vi "Main.vi"(8 "error":errorcluster) -> (0 "Error out":errorcluster)   [LabVIEW 2018, in "GUI3.lvclass"]
uses:
  GUI3.lvclass
  Public Controls/TestInfo.ctl
  S6/S6.lvclass
  S5/S5.lvclass
panel:
  in  "Tab Control":enum32{"TESTS SCREEN"}(tab)
  out "S5 Valves":bool[](array[boolean])
  out "EC_PTEST_DELTA_MAX":dbl format="%.2f psig"
  in  "S5AckAlarm":bool
  out "PRESSURE PT1_S6":dbl(knob) caption="PRESSURE PT1" scale=0.0..400.0
  out "ELAPSED TIME 5":dbl caption="REMAINING STATE TIME" format="%<%H:%M:%S>t"
  out "IsLidLocked_S5":bool caption="IsLidLocked"
  in  "SN_S5":string caption="SN"
  in  "S5Start":bool
  in  "ABORT_S5":bool
  out "TEST STOPPED AT:":string
  out "TEST STARTED AT:":string
  out "PRESSURE PT531":dbl(knob) scale=0.0..400.0
  out "PRESSURE PT521":dbl(knob) scale=0.0..400.0
  out "TEST RESULT_S5":string caption="TEST RESULT"
  out "TEST STATE_S5":string caption="TEST STATE"
  out "Pressure vs Time Plot 3":waveform(dbl)[](graph)
  out "TEST STATUS 5":string caption="TEST STATUS"
  in  "Select Test Type_S5":string(combo) caption="Test Type"
  out "S6 Valves":bool[](array[boolean])
  out "EC_PTEST_DELTA_MAX":dbl format="%.2f psig"
  in  "S6AckAlarm":bool
  out "PRESSURE PT1_S5":dbl(knob) caption="PRESSURE PT1" scale=0.0..400.0
  out "ELAPSED TIME 6":dbl caption="REMAINING STATE TIME" format="%<%H:%M:%S>t"
  out "IsLidLocked_S6":bool caption="IsLidLocked"
  in  "SN_S6":string caption="SN"
  in  "S6Start":bool
  in  "ABORT_S6":bool
  out "TEST STOPPED AT:":string
  out "TEST STARTED AT:":string
  out "PRESSURE PT631":dbl(knob) scale=0.0..400.0
  out "PRESSURE PT621":dbl(knob) scale=0.0..400.0
  out "TEST RESULT_S6":string caption="TEST RESULT"
  out "TEST STATE_S6":string caption="TEST STATE"
  out "Pressure vs Time Plot 4":waveform(dbl)[](graph)
  out "TEST STATUS 6":string caption="TEST STATUS"
  in  "Select Test Type_S6":string(combo) caption="Test Type"
  # "This template is for the Simple State Machine design pattern.\n\nSee the block diagram for more information on how to use this template."
  # "STATION #5"
  # "STATION #6"
  # "LoP"
  # "HiP"
  # "Z3"
  # "Z2"
  # "Lid Ext"
  # "LoP"
  # "HiP"
  # "Z3"
  # "Z2"
  # "Lid Ext"
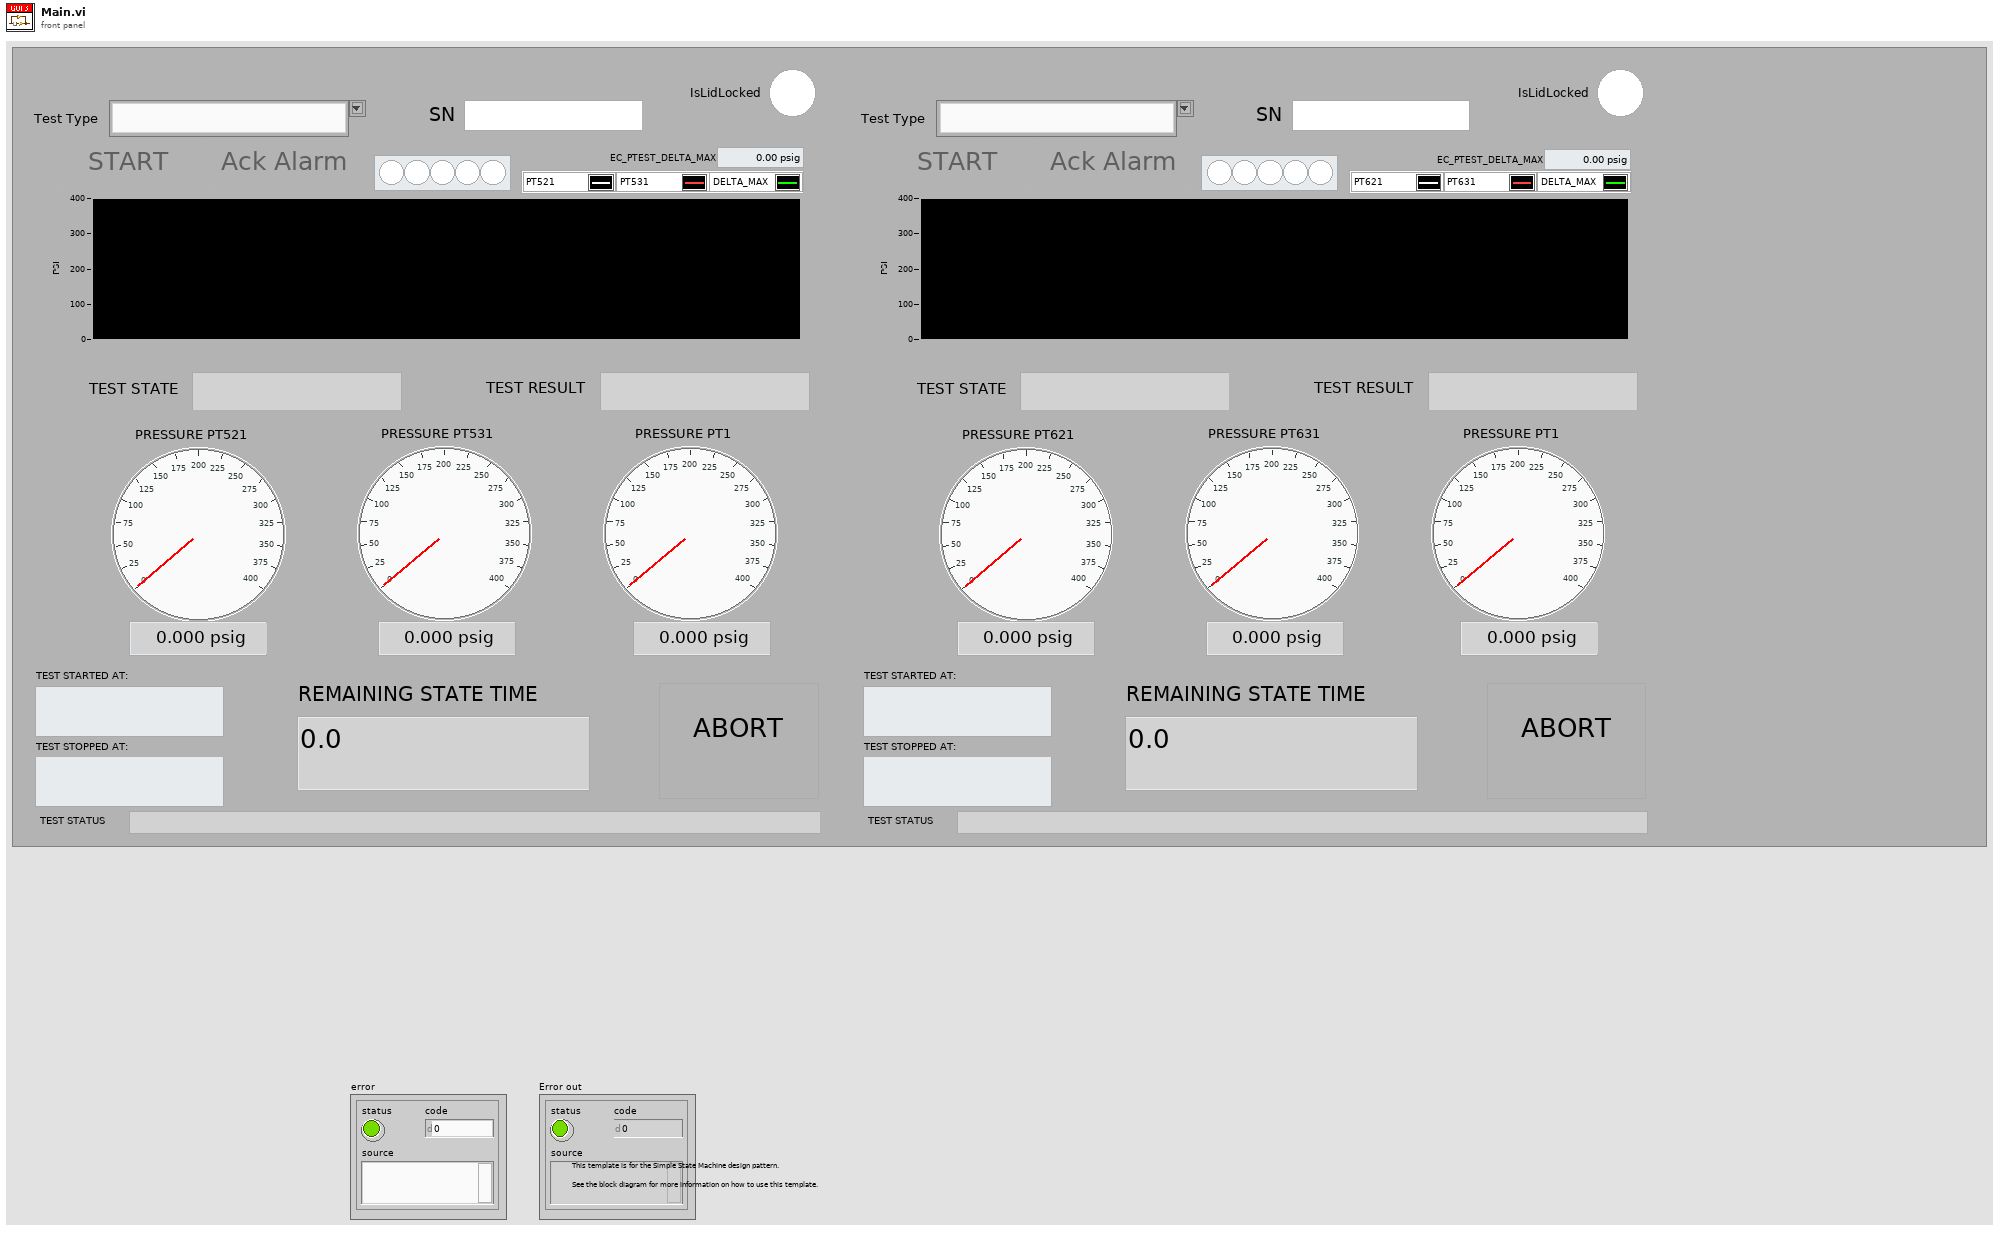
[diagram p1: front panel]
types:
  T1 = enum8{"Enabled", "Disabled", "Disabled and Grayed Out"}
  T2 = typedef "GUI3.lvclass/State.ctl" = enum16{"Initialize", "S5Alarm", "S6Alarm", "S5EndOfTest", "S6EndOfTest", "Monitor", "Error", "Exit"}
  T3 = typedef "GUI3.lvclass/TestInfo.ctl" = cluster{"TestType":string, "SN":string}
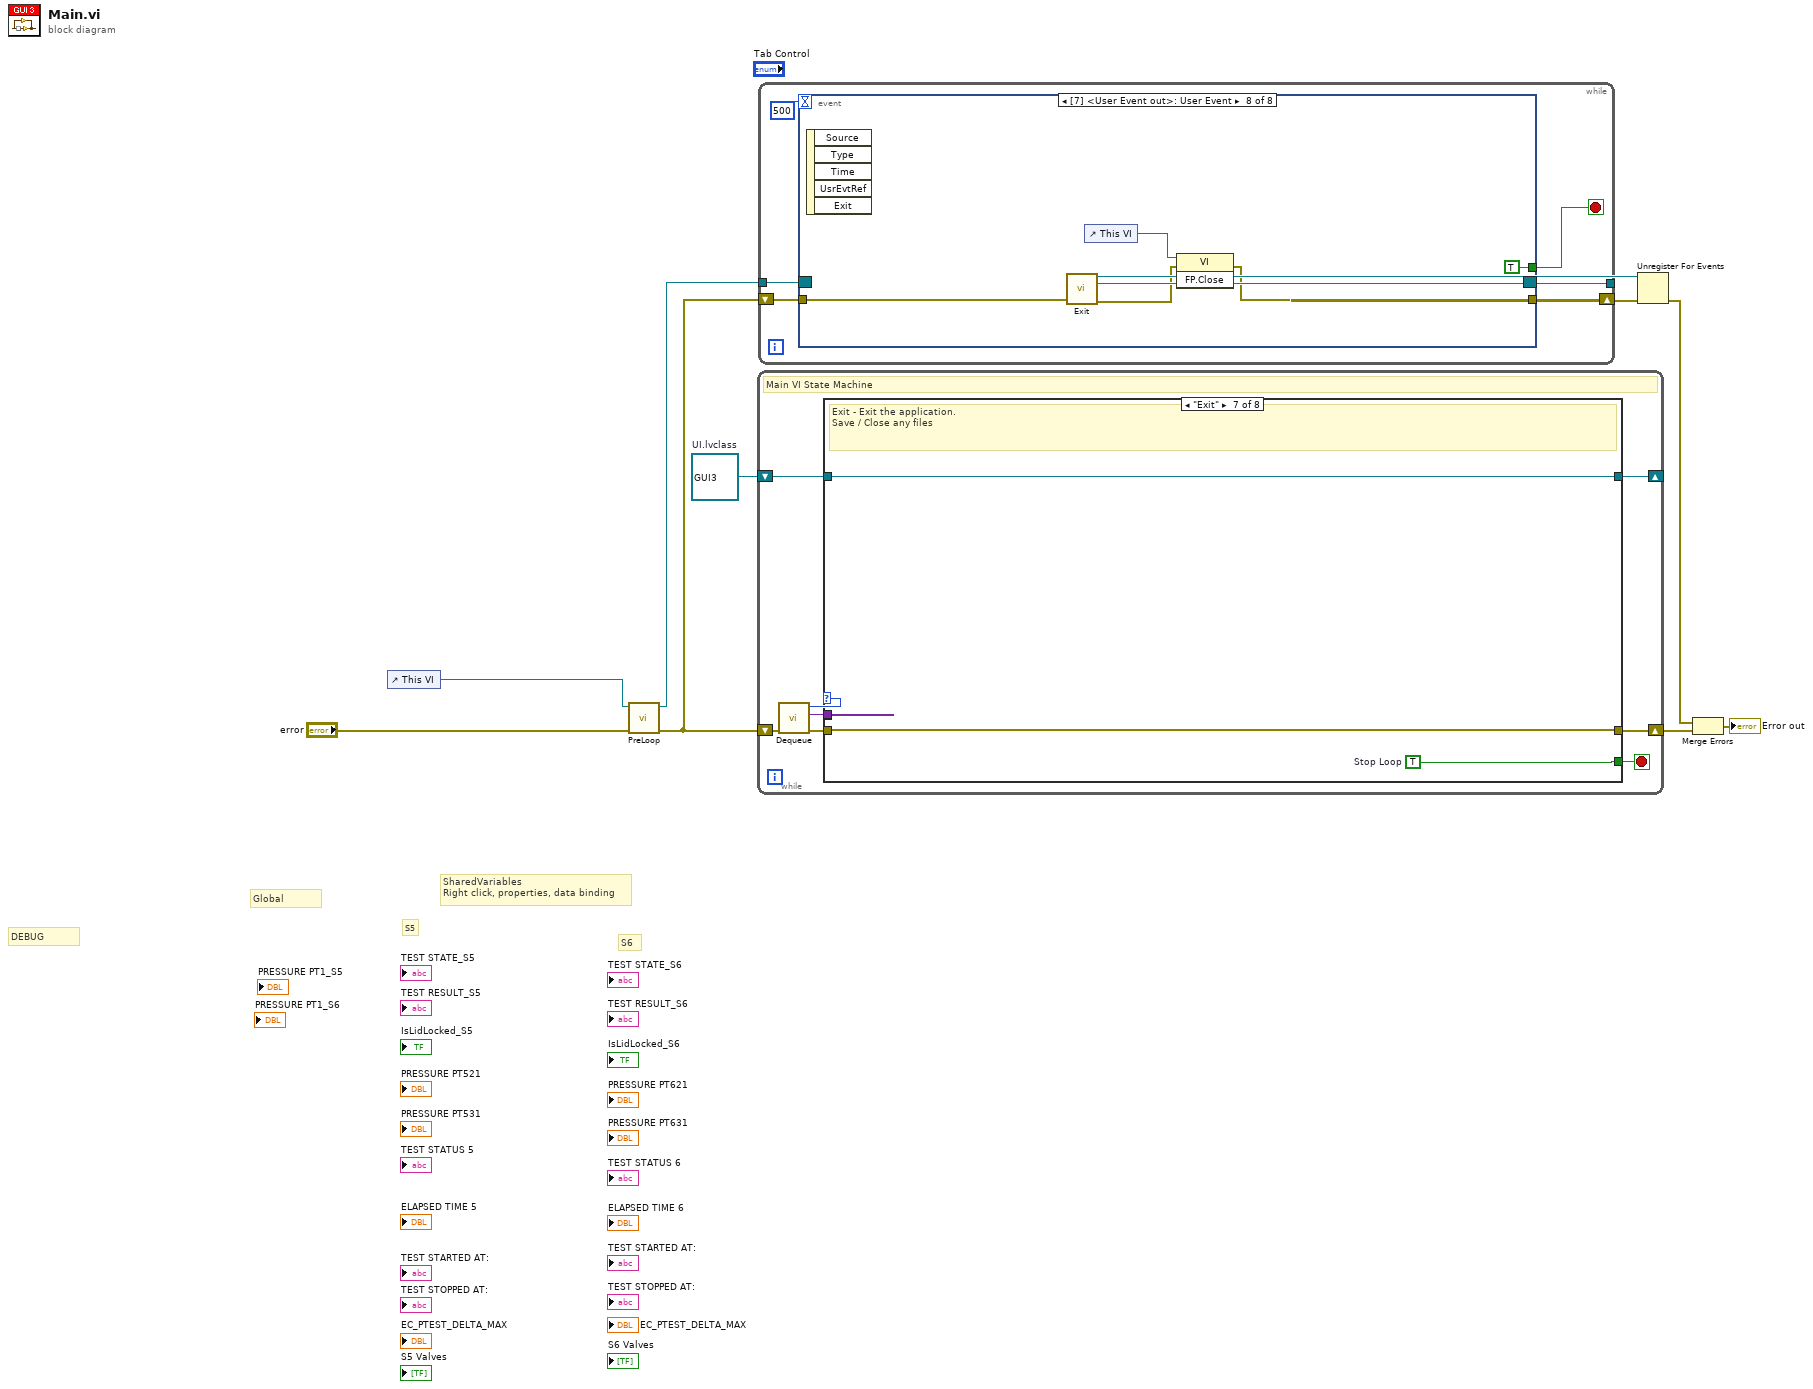
[diagram p0: block diagram]
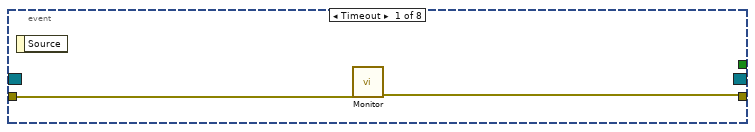
[diagram p2: hidden frame]
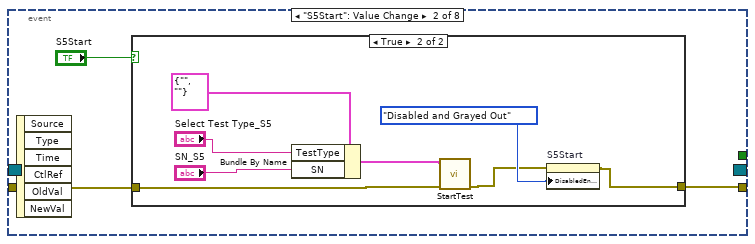
[diagram p3: hidden frame]
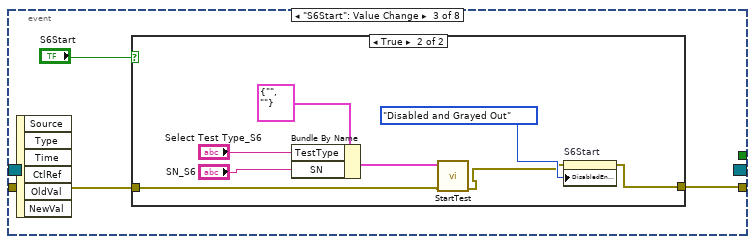
[diagram p5: hidden frame]
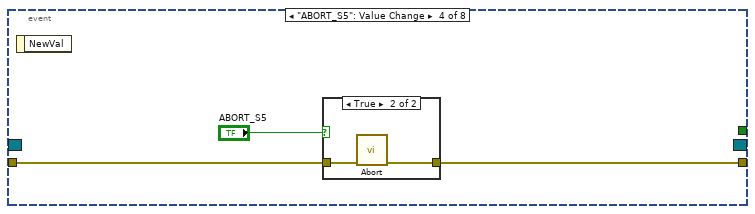
[diagram p7: hidden frame]
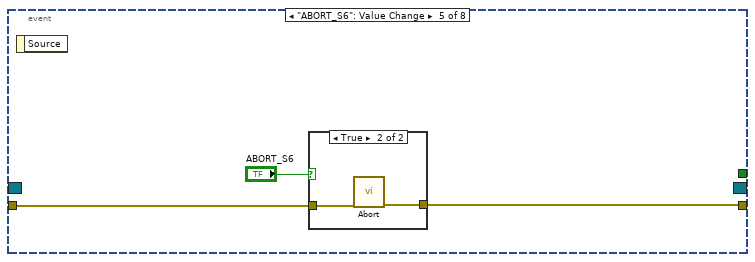
[diagram p9: hidden frame]
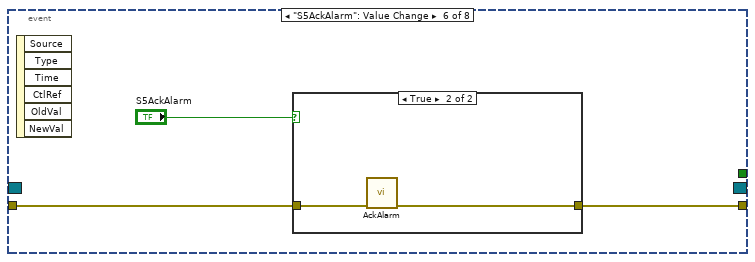
[diagram p11: hidden frame]
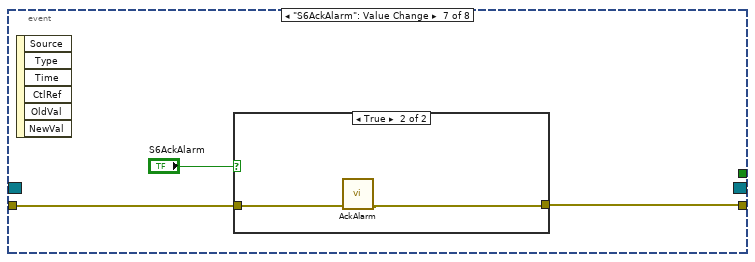
[diagram p13: hidden frame]
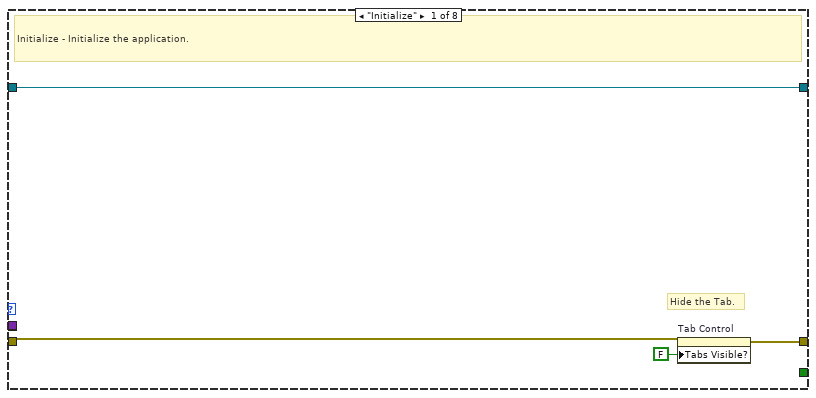
[diagram p15: hidden frame]
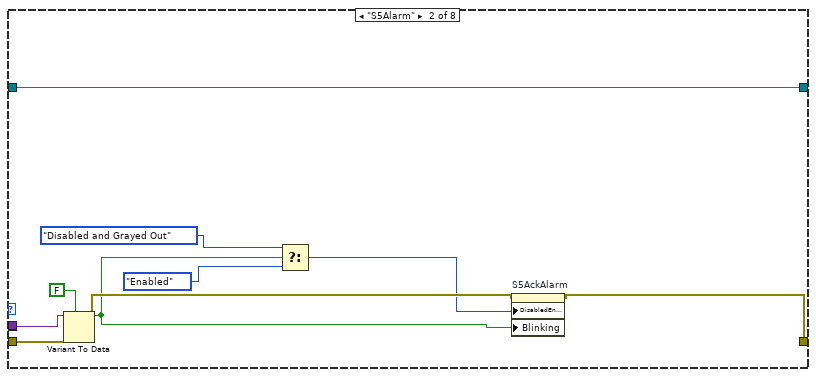
[diagram p16: hidden frame]
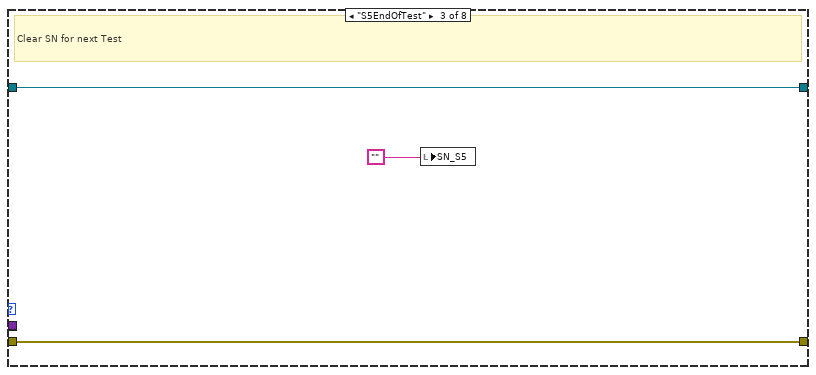
[diagram p17: hidden frame]
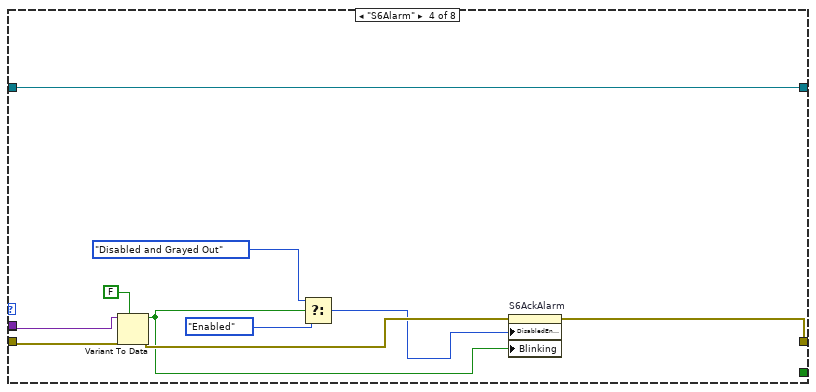
[diagram p18: hidden frame]
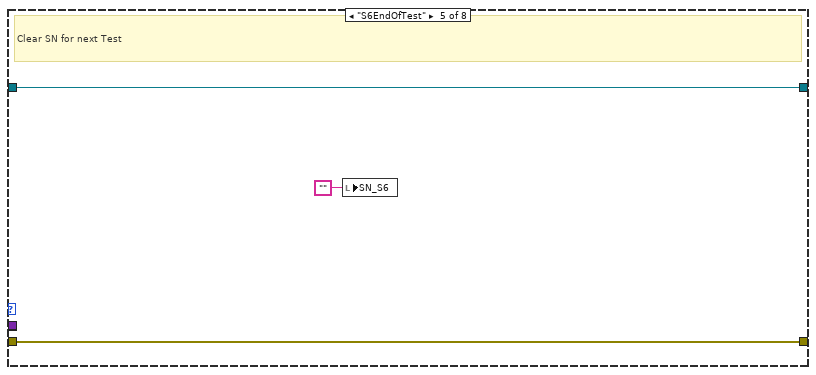
[diagram p19: hidden frame]
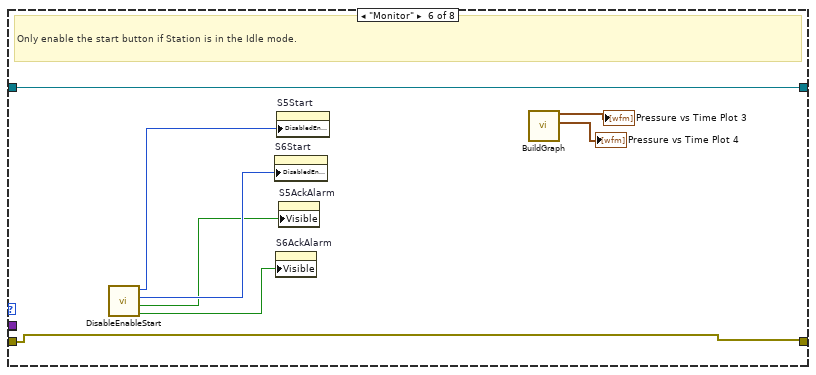
[diagram p20: hidden frame]
diagram:
  w10 = refnum<class "GUI3.lvclass"> refnum  # UI.lvclass
  # "Global"
  # "S6"
  # "DEBUG"
  # "S5"
  # "SharedVariables\nRight click, properties, data binding"
  n1 = control-ref of="This VI"() -> (w1:refnum<vi>)
  n2 = call "PreLoop.vi"("error in"="error", "VI Ref"=w1) -> ("error out"=w9:errorcluster, "Event Out"=w3:refnum<event-registration>)  [unwired: 8 in]
  n3 = while {
    shift-right: [w18] -> w6
    shift-left: w9 -> [w14]
    shift-right: [w15] -> _
    shift-left: w10 -> [w16]
    stop <- w17 stop-if-true
    # "Main VI State Machine"
    n4 = call "Dequeue.vi"("error in"=w14) -> ("error out"=w13:errorcluster, "Data"=w11:variant, "State"=w12:T2)  [unwired: 8 in]
    n5 = case shown="\"Exit\"" w12 {
      tunnel: [_ _ _ _ _ _ w59 _] -> w17
      tunnel: w13 -> [w19 w31 w35 w41 w48 w49 w57 w65]
      tunnel: [w20 w25 w35 w36 w48 w49 w57 w61] -> w18
      tunnel: w16 -> [w22 w32 w34 w45 w47 w56 w58 w68]
      tunnel: [w22 w32 w34 w45 w47 w56 w58 w68] -> w15
      tunnel: w11 -> [_ w30 _ w40 _ _ _ w64]
      tunnel: w11 -> [_ _ _ _ _ _ _ _]
      frame "Initialize" {
        # "Hide the Tab."
        # "Initialize - Initialize the application."
        n6 = property on="Tab Control" class="TabCtl (strict)"(error in=w19, "Tabs Visible?"=FALSE) -> (error out=w20:errorcluster)  [unwired: 1 in, 1 out]
      }
      frame "S5Alarm" {
        n7 = Variant To Data(error in=w31, type=FALSE, Variant=w30) -> (data=w23:bool, error out=w26:errorcluster)
        n8 = Select(t=T1."Disabled and Grayed Out" ("Disabled"), s=w23, f=T1."Enabled" ("Disabled")) -> (s? t:f=w24:T1)
        n9 = property on="S5AckAlarm" class="Bool"(error in=w26, "DisabledEnum"=w24, "Blinking"=w23) -> (error out=w25:errorcluster)  [unwired: 1 in, 1 out]
      }
      frame "S5EndOfTest" {
        # "Clear SN for next Test"
        n10 = local write "SN_S5"("" ("SN")) -> ()
      }
      frame "S6Alarm" {
        n11 = Variant To Data(error in=w41, type=FALSE, Variant=w40) -> (data=w37:bool, error out=w39:errorcluster)
        n12 = Select(t=T1."Disabled and Grayed Out" ("Disabled"), s=w37, f=T1."Enabled" ("Disabled")) -> (s? t:f=w38:T1)
        n13 = property on="S6AckAlarm" class="Bool"(error in=w39, "DisabledEnum"=w38, "Blinking"=w37) -> (error out=w36:errorcluster)  [unwired: 1 in, 1 out]
      }
      frame "S6EndOfTest" {
        # "Clear SN for next Test"
        n14 = local write "SN_S6"("") -> ()
      }
      frame "Monitor" {
        # "Only enable the start button if Station is in the Idle mode."
        n15 = call "DisableEnableStart.vi"() -> ("S6AckVisable"=w50:bool, "S5AckVisable"=w52:bool, "Station6"=w55:T1, "Station5"=w51:T1)  [unwired: 8 in]
        n16 = property on="S6Start" class="Bool"("DisabledEnum"=w55) -> ()  [unwired: 2 in, 2 out]
        n17 = property on="S6AckAlarm" class="Bool"("Visible"=w50) -> ()  [unwired: 2 in, 2 out]
        n18 = property on="S5Start" class="Bool"("DisabledEnum"=w51) -> ()  [unwired: 2 in, 2 out]
        n19 = property on="S5AckAlarm" class="Bool"("Visible"=w52) -> ()  [unwired: 2 in, 2 out]
        n20 = call "BuildGraph.vi"() -> ("S6"=→"Pressure vs Time Plot 4":waveform(dbl)[], "S5"=→"Pressure vs Time Plot 3":waveform(dbl)[])  [unwired: 10 in]
      }
      frame "Exit" {
        w59 = TRUE  # Stop Loop
        # "Exit - Exit the application.\nSave / Close any files"
      }
      frame "Error" {
        n21 = Variant To Data(error in=w65, type=errorcluster {"status"=FALSE, "code"=0, "source"=""} ("error out"), Variant=w64) -> (data=w66:errorcluster, error out=w62:errorcluster)
        n22 = Unbundle By Name(w66) -> ("code"=w60:i32, "source"=w63:string)
        n23 = case shown="Default" w60 {
          tunnel: w63 -> [_ w71]
          tunnel: w62 -> [w69 w73]
          tunnel: [w69 w73] -> w61
          frame 1 {
            # "Error talking to other modules. \n\nIgnore. If testing by itself."
          }
          frame Default {
            n24 = Concatenate Strings("Error on GUI" ("message"), w71) -> (w70:string)
            n25 = One Button Dialog(message=w70) -> ()  [unwired: 1 in, 1 out]
          }
        }
      }
    }
  }
  n26 = while {
    shift-right: [w77] -> w8
    shift-left: w9 -> [w79]
    tunnel: [w76] -> w7
    tunnel: w3 -> [w74]
    stop <- w78 stop-if-true
    n27 = event shown="[7] <User Event out>: User Event" {
      selector: w74 -> [_ _ _ _ _ _ _ _]
      dyn-events: [_ _ _ _ _ _ _ _] -> w76
      timeout: 500 -> [_ _ _ _ _ _ _ _]
      tunnel: w79 -> [w81 w84 w96 w108 w114 w120 w125 w134]
      tunnel: [w80 w83 w95 w107 w112 w119 w124 w130] -> w77
      tunnel: [_ _ _ _ _ _ _ TRUE] -> w78
      event Timeout {
        n28 = event-data() -> ()  [unwired: 1 in, 1 out]
        n29 = call "Monitor.vi"("error in"=w81) -> ("error out"=w80:errorcluster)  [unwired: 10 in]
      }
      event "S5Start": Value Change {
        n30 = event-data() -> ()  [unwired: 1 in, 6 out]
        n31 = case shown="True" "S5Start" {
          tunnel: w84 -> [w85 w87]
          tunnel: [w85 w89] -> w83
          frame False {
          }
          frame True {
            n32 = Bundle By Name(cluster=T3 {"TestType"="", "SN"=""}, "TestType"="Select Test Type_S5", "SN"="SN_S5") -> (w88:T3)
            n33 = call "StartTest.vi"("error in"=w87, "TestInfo"=w88) -> ("error out"=w86:errorcluster)  [unwired: 9 in]
            n34 = property on="S5Start" class="Bool"(error in=w86, "DisabledEnum"=T1."Disabled and Grayed Out" ("Disabled")) -> (error out=w89:errorcluster)  [unwired: 1 in, 1 out]
          }
        }
      }
      event "S6Start": Value Change {
        n35 = event-data() -> ()  [unwired: 1 in, 6 out]
        n36 = case shown="True" "S6Start" {
          tunnel: w96 -> [w97 w99]
          tunnel: [w97 w102] -> w95
          frame False {
          }
          frame True {
            n37 = Bundle By Name(cluster=T3 {"TestType"="", "SN"=""}, "TestType"="Select Test Type_S6", "SN"="SN_S6") -> (w100:T3)
            n38 = call "StartTest.vi"("error in"=w99, "TestInfo"=w100) -> ("error out"=w98:errorcluster)  [unwired: 9 in]
            n39 = property on="S6Start" class="Bool"(error in=w98, "DisabledEnum"=T1."Disabled and Grayed Out" ("Disabled")) -> (error out=w102:errorcluster)  [unwired: 1 in, 1 out]
          }
        }
      }
      event "ABORT_S5": Value Change {
        n40 = event-data() -> ()  [unwired: 1 in, 1 out]
        n41 = case shown="True" "ABORT_S5" {
          tunnel: w108 -> [w109 w111]
          tunnel: [w109 w110] -> w107
          frame False {
          }
          frame True {
            n42 = call "Abort.vi"("error in"=w111) -> ("error out"=w110:errorcluster)  [unwired: 10 in]
          }
        }
      }
      event "ABORT_S6": Value Change {
        n43 = event-data() -> ()  [unwired: 1 in, 1 out]
        n44 = case shown="True" "ABORT_S6" {
          tunnel: w114 -> [w115 w117]
          tunnel: [w115 w116] -> w112
          frame False {
          }
          frame True {
            n45 = call "Abort.vi"("error in"=w117) -> ("error out"=w116:errorcluster)  [unwired: 10 in]
          }
        }
      }
      event "S5AckAlarm": Value Change {
        n46 = event-data() -> ()  [unwired: 1 in, 6 out]
        n47 = case shown="True" "S5AckAlarm" {
          tunnel: w120 -> [w121 w123]
          tunnel: [w121 w122] -> w119
          frame False {
          }
          frame True {
            n48 = call "AckAlarm.vi"("error in"=w123) -> ("error out"=w122:errorcluster)  [unwired: 10 in]
          }
        }
      }
      event "S6AckAlarm": Value Change {
        n49 = event-data() -> ()  [unwired: 1 in, 6 out]
        n50 = case shown="True" "S6AckAlarm" {
          tunnel: w125 -> [w127 w129]
          tunnel: [w127 w128] -> w124
          frame False {
          }
          frame True {
            n51 = call "AckAlarm.vi"("error in"=w129) -> ("error out"=w128:errorcluster)  [unwired: 10 in]
          }
        }
      }
      event User Event {
        n52 = event-data() -> ()  [unwired: 1 in, 5 out]
        n53 = call "Exit.vi"("error in"=w134) -> ("error out"=w131:errorcluster)  [unwired: 10 in]
        n54 = control-ref of="This VI"() -> (w132:refnum<vi>)
        n55 = invoke class="VI" method="FP.Close"(reference=w132, error in=w131) -> (error out=w130:errorcluster)  [unwired: 1 in, 2 out]
      }
    }
  }
  n56 = Unregister For Events(event registration refnum=w7, error in=w8) -> (error out=w5:errorcluster)
  n57 = Merge Errors(w5, w6) -> (→"Error out":errorcluster)
